vi "Visa Names Unique.vi"(11 "VISA resource names In":refnum<visa-resource-name>[](array[refnum])=["GPIB0::4::INSTR", "GPIB0::5::INSTR", "GPIB0::5::INSTR", "GPIB0::14::INSTR", "GPIB0::16::INSTR", "GPIB0::16::INSTR", "GPIB0::17::INSTR"]) -> (3 "Unique VISA resource namesOut":refnum<visa-resource-name>[](array[refnum]))   [LabVIEW 2024]
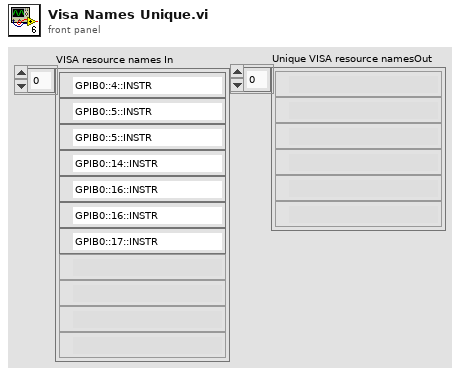
[diagram p1: front panel]
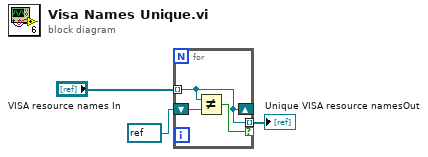
[diagram p0: block diagram]
diagram:
  n1 = for {
    tunnel: "VISA resource names In" -> [w5] mode=indexing
    tunnel: [w5] -> w2 mode=indexing if=w6
    shift-right: [w5] -> _
    shift-left: refnum<visa-resource-name> refnum ("VISA resource name") -> [w4]
    n2 = Not Equal?(x=w5, y=w4) -> (x != y?=w6:bool)
  }
  "Unique VISA resource namesOut" <- w2
